vi "Simulation Kobuki Sensors.vi"(8 "error in":errorcluster, 9 "Feedback Input":T1, 10 "Robot":T2, 11 "simulator":T8={"configuration"={"maxTime"=5.0, "enableVisualization"=TRUE, "Environment Definition"=path "simulation configuration.ini", "Record Location"=path "Simulation Record.xml", "autograde?"=TRUE, "interactive?"=FALSE, "Feedback Mode"=enum."debug navigation", "Robot State Charts"=[path "C:/Users/blueuser/Desktop/Robo Sim Berkley/cpsgrader-release-0.4/Simulators/EECS149lab/src/LabVIEW/statechart/Simulation Statechart.vi"], "statechart"=path "iRobot Navigation State Machine.vi"}, "Statechart\ndisplay"=refnum, "first step?"=FALSE, "Robots Simulation Statecharts"=[], "Robots"=[]}) -> (0 "error out":errorcluster, 1 "Feedback Output":T1, 2 "sensors":T3 {"Kobuki Sensors"."Charger Source" items=["DISCHARGING"=0, "DOCKING_CHARGED"=2, "DOCKING_CHARGING"=6, "ADAPTER_CHARGED"=18, "ADAPTER_CHARGING"=22]; "accelerometer"."z axis (g)" format="%.3f"; "accelerometer"."y axis (g)" format="%.3f"; "accelerometer"."x axis (g)" format="%.3f"}, 3 "simulator":T8={"configuration"={"maxTime"=5.0, "enableVisualization"=TRUE, "Environment Definition"=path "simulation configuration.ini", "Record Location"=path "Simulation Record.xml", "autograde?"=TRUE, "interactive?"=FALSE, "Feedback Mode"=enum."debug navigation", "Robot State Charts"=[path "C:/Users/blueuser/Desktop/Robo Sim Berkley/cpsgrader-release-0.4/Simulators/EECS149lab/src/LabVIEW/statechart/Simulation Statechart.vi"], "statechart"=path "iRobot Navigation State Machine.vi"}, "Statechart\ndisplay"=refnum, "first step?"=FALSE, "Robots Simulation Statecharts"=[], "Robots"=[]})   [LabVIEW 2015]
doc: "Simulates iRobot sensors. Automatically accumulates distance and angle."
uses:
  Simulator.ctl
  <instrlib>/DC Motor Controller/HAIOL/DC Motor Controller.lvclass
  CyberSim interface/Simulation Configuration.ctl
  autograder/feedbackMode.ctl
  Multi Bot Code/RobotData.ctl
  shared/Sensors.ctl
  shared/Accelerometer.ctl
  Kobuki/KobukiSensors.ctl
  Kobuki/Kobuki Bumps and WheelDrops.ctl
  Kobuki/Kobuki Buttons.ctl
  Multi Bot Code/Sim Sensors Feedback.ctl
  <vilib>/Analysis/coordinate.llb/Angle Units.ctl
  <vilib>/Analysis/coordinate.llb/Wrap Angle (scalar).vi
  <vilib>/Analysis/BLAS.llb/dnrm2 - Vector 2-Norm (DBL).vi
  <resource>/objmgr/LVODE.rc
  <vilib>/Analysis/NI_AALBLAS.lvlib
  <vilib>/robotics/Kinematics/NI_Kinematics.lvlib
  <vilib>/Analysis/NI_AAL_Angle.lvlib
panel:
  out "size(s)":i32
  out "Roll":dbl
  out "pitch":dbl
  out "Yaw":dbl
  # "Electrical: charging, battery, OI mode"
  # "Sensors: bump, cliff, button, wheel drop"
  # "Motors:"
  # "Inertia"
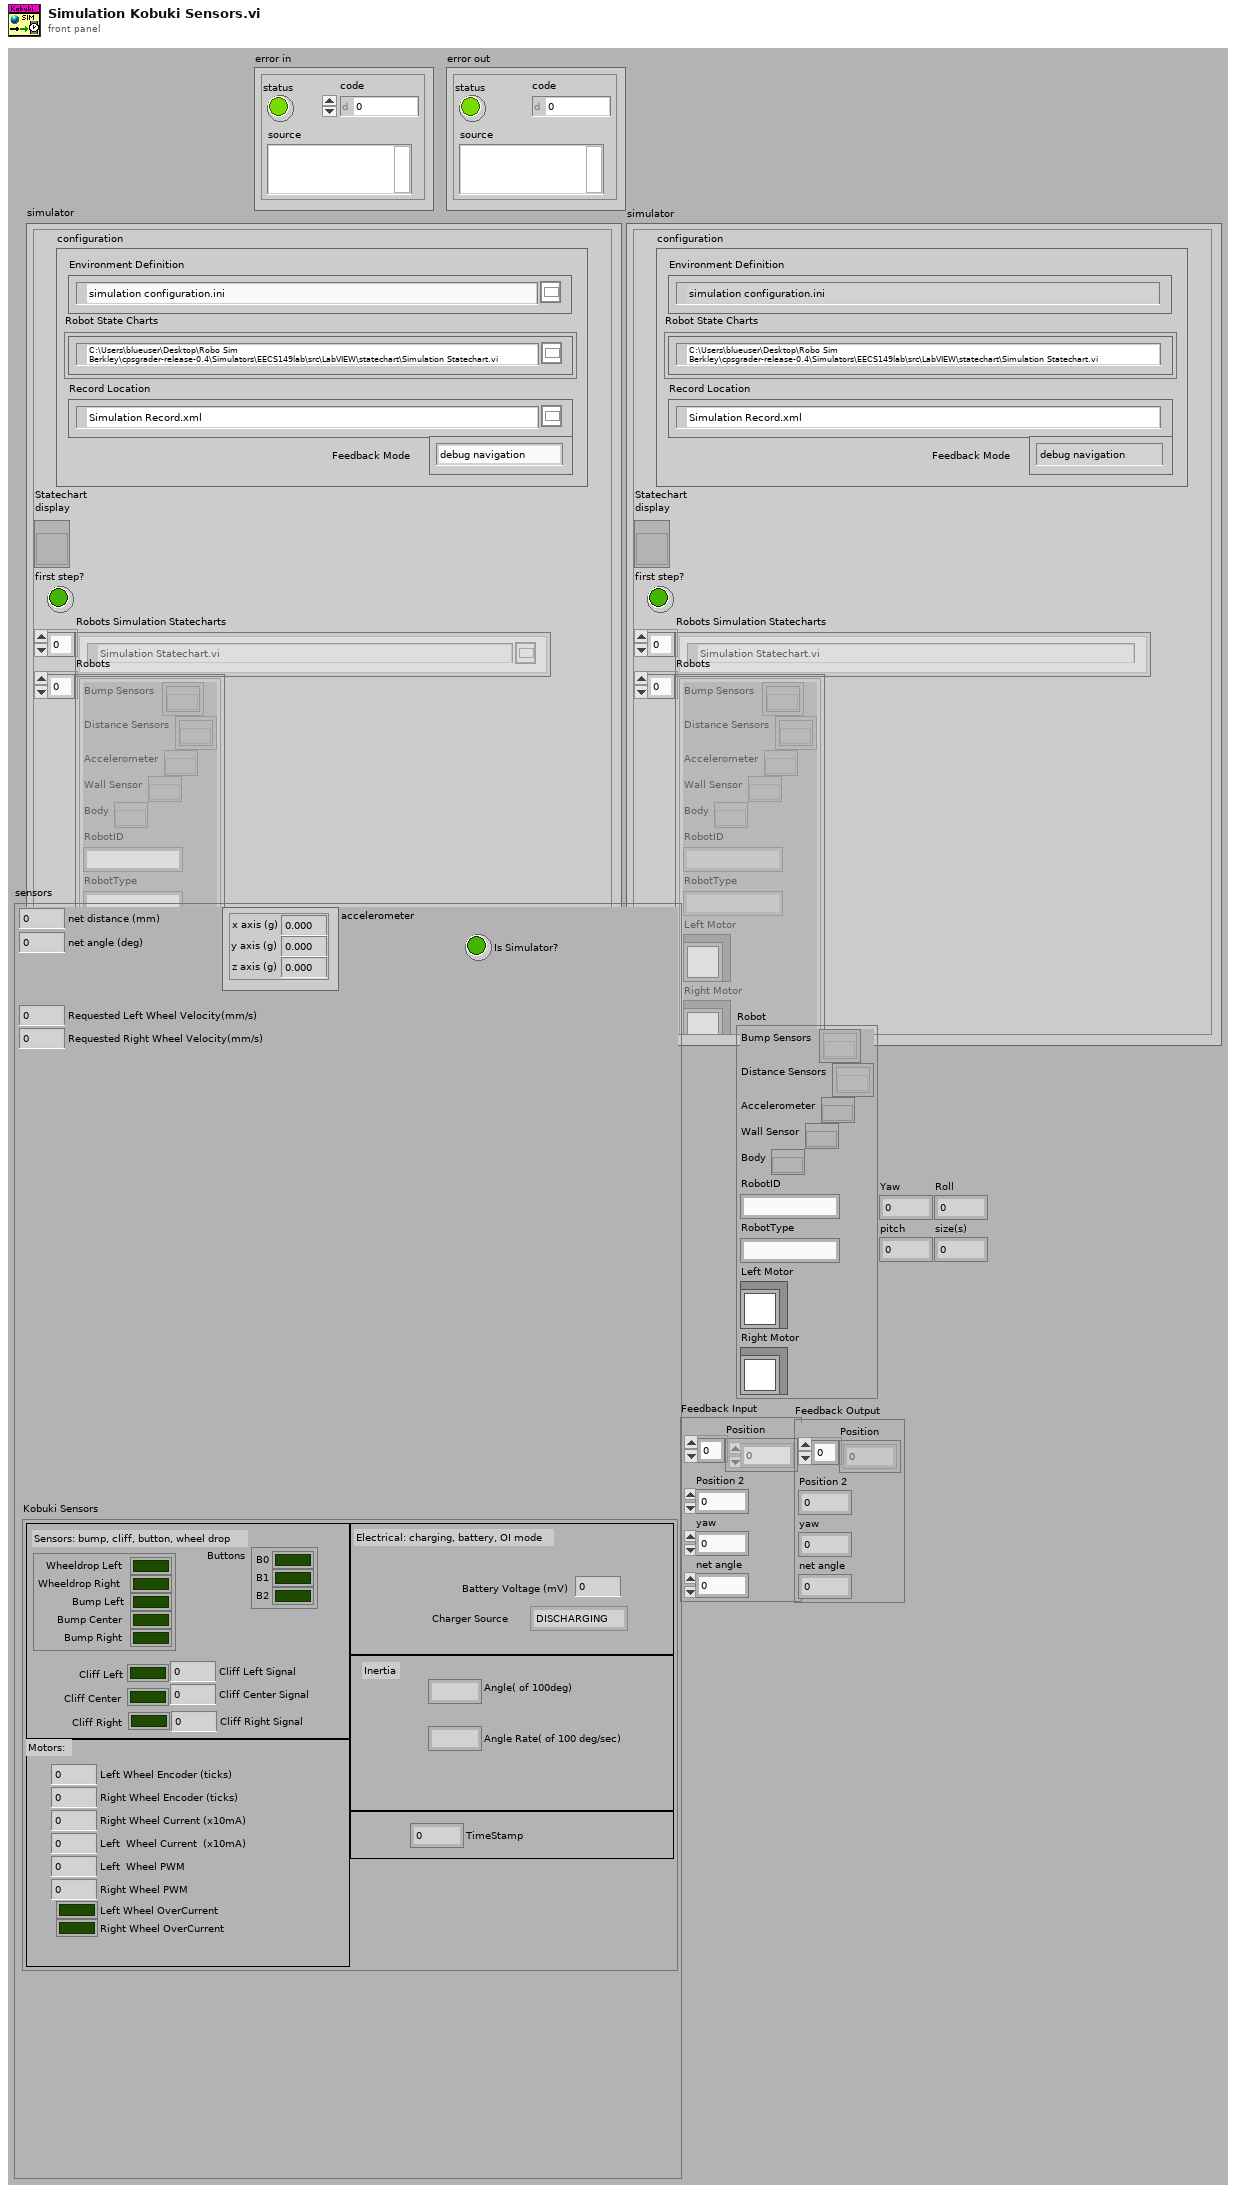
[diagram p1: front panel]
types:
  T1 = typedef "Sim Sensors Feedback.ctl" = cluster{"Position":sgl[], "Position 2":dbl, "yaw":dbl, "net angle":dbl}
  T2 = typedef "RobotData.ctl" = cluster{"Bump Sensors":refnum<k20>[], "Distance Sensors":refnum<k20>[], "Accelerometer":refnum<k20>, "Wall Sensor":refnum<k20>, "Body":refnum<k20>, "RobotID":string, "RobotType":string, "Left Motor":refnum<class "DC Motor Controller.lvclass">, "Right Motor":refnum<class "DC Motor Controller.lvclass">}
  T3 = typedef "Sensors.ctl" = cluster{"net distance (mm)":i32, "net angle (deg)":i32, "accelerometer":T4, "Is Simulator?":bool, "Kobuki Sensors":T5, "Requested Left Wheel Velocity(mm/s)":i32, "Requested Right Wheel Velocity(mm/s)":i32}
  T4 = typedef "Accelerometer.ctl" = cluster{"x axis (g)":dbl, "y axis (g)":dbl, "z axis (g)":dbl}
  T5 = typedef "KobukiSensors.ctl" = cluster{"Bumps + Wheel Drops":T6, "Cliff Left":bool, "Cliff Center":bool, "Cliff Right":bool, "Cliff Left Signal":u16, "Cliff Center Signal":u16, "Cliff Right Signal":u16, "Buttons":T7, "Left Wheel Encoder (ticks)":u16, "Right Wheel Encoder (ticks) ":u16, "Left  Wheel PWM":i8, "Right Wheel PWM":i8, "Left Wheel OverCurrent":bool, "Right Wheel OverCurrent ":bool, "Right Wheel Current (x10mA)":i16, "Left  Wheel Current  (x10mA)":i16, "TimeStamp":u16, "Battery Voltage (mV)":i16, "Angle( of 100deg)":i16, "Angle Rate( of 100 deg/sec)":i16, "Charger Source ":i8}
  T6 = typedef "Kobuki Bumps and WheelDrops.ctl" = cluster{"Wheeldrop Left":bool, "Wheeldrop Right":bool, "Bump Left":bool, "Bump Center":bool, "Bump Right":bool}
  T7 = typedef "Kobuki Buttons.ctl" = cluster{"B0":bool, "B1":bool, "B2":bool}
  T8 = typedef "Simulator.ctl" = cluster{"configuration":T9, "Statechart\ndisplay":refnum<vi>, "first step?":bool, "Robots Simulation Statecharts":path[], "Robots":T2[]}
  T9 = typedef "Simulation Configuration.ctl" = cluster{"maxTime":sgl, "enableVisualization":bool, "Environment Definition":path, "Record Location":path, "autograde?":bool, "interactive?":bool, "Feedback Mode":T10, "Robot State Charts":path[], "statechart":path}
  T10 = typedef "feedbackMode.ctl" = enum32{"debug navigation", "debug hill climb", "autograde navigation", "autograde hill climb"}
  T11 = typedef "NI_AAL_Angle.lvlib/Angle Units.ctl" = i32
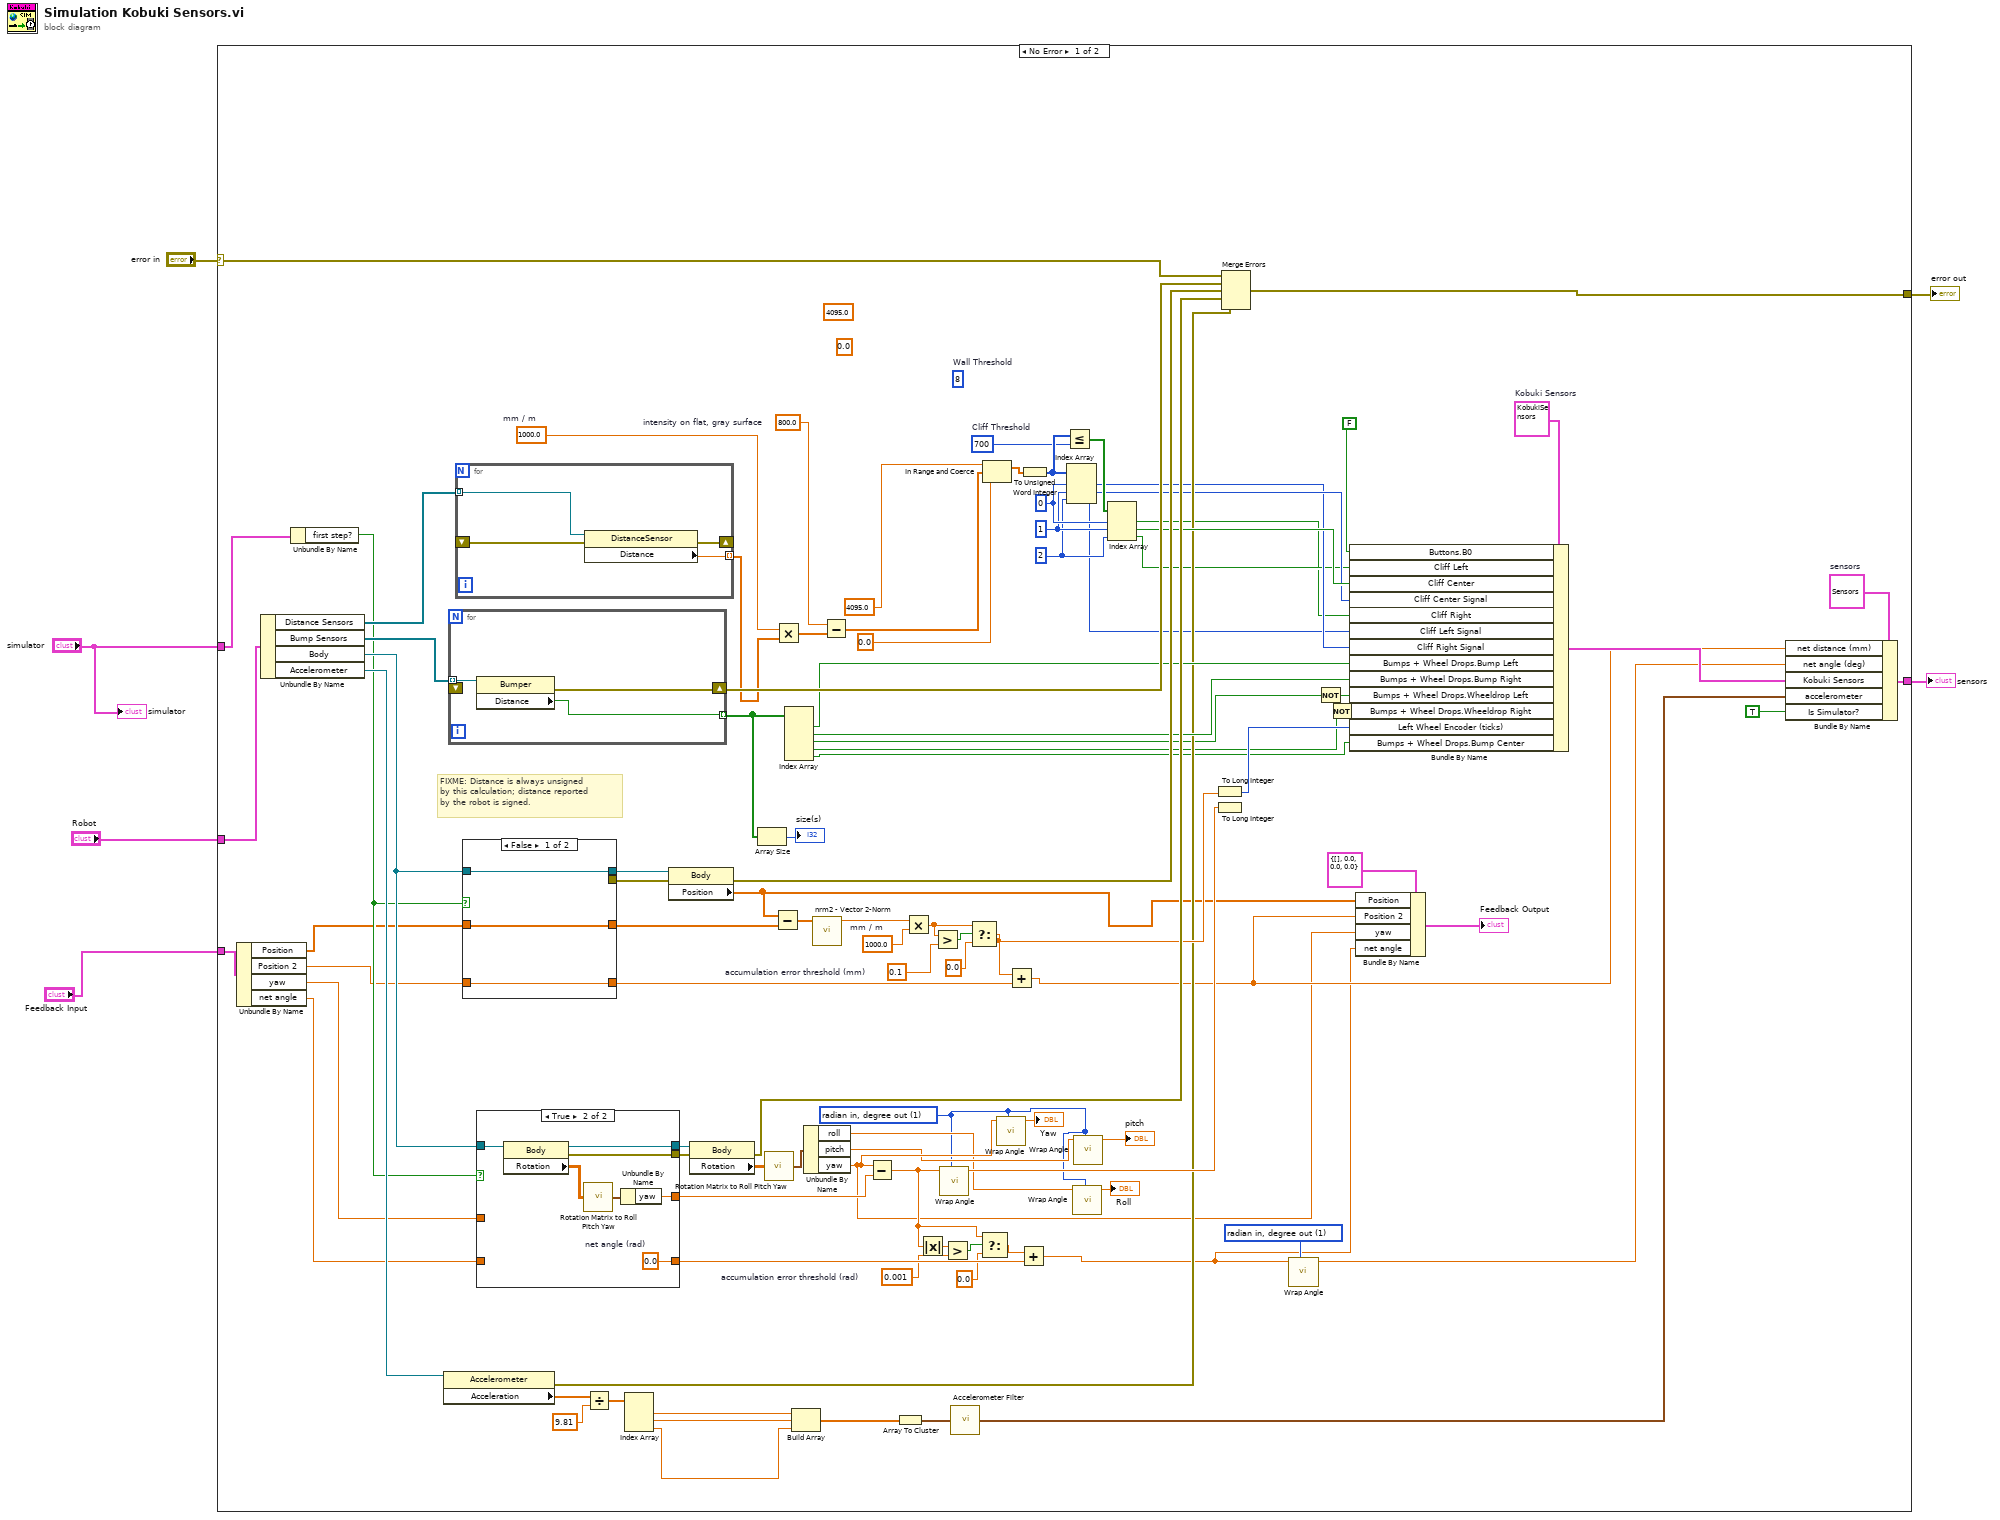
[diagram p0: block diagram]
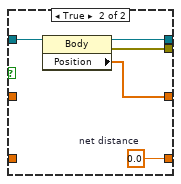
[diagram p3: hidden frame]
diagram:
  n1 = case shown="No Error" "error in" {
    selector: "error in" -> [w71 w134]
    tunnel: [w76 _] -> w6
    tunnel: "simulator" -> [w61 _]
    tunnel: [w72 w134] -> w4
    tunnel: "Robot" -> [w62 _]
    tunnel: "Feedback Input" -> [w59 _]
    frame No Error {
      w14 = T11 1 items=["radian in, radian out", "radian in, degree out", "degree in, degree out", "degree in, radian out"] ("angle units")
      w29 = 0.001  # accumulation error threshold (rad)
      w40 = 0.1  # accumulation error threshold (mm)
      w45 = 1000.0  # mm / m
      w24 = 2 ("index")
      w65 = 1 ("index")
      w66 = 0 ("index")
      w77 = T3 {"net distance (mm)"=0, "net angle (deg)"=0, "accelerometer"={"x axis (g)"=0.0, "y axis (g)"=0.0, "z axis (g)"=0.0}, "Is Simulator?"=FALSE, "Kobuki Sensors"={"Bumps + Wheel Drops"={"Wheeldrop Left"=FALSE, "Wheeldrop Right"=FALSE, "Bump Left"=FALSE, "Bump Center"=FALSE, "Bump Right"=FALSE}, "Cliff Left"=FALSE, "Cliff Center"=FALSE, "Cliff Right"=FALSE, "Cliff Left Signal"=0, "Cliff Center Signal"=0, "Cliff Right Signal"=0, "Buttons"={"B0"=FALSE, "B1"=FALSE, "B2"=FALSE}, "Left Wheel Encoder (ticks)"=0, "Right Wheel Encoder (ticks) "=0, "Left  Wheel PWM"=0, "Right Wheel PWM"=0, "Left Wheel OverCurrent"=FALSE, "Right Wheel OverCurrent "=FALSE, "Right Wheel Current (x10mA)"=0, "Left  Wheel Current  (x10mA)"=0, "TimeStamp"=0, "Battery Voltage (mV)"=0, "Angle( of 100deg)"=0, "Angle Rate( of 100 deg/sec)"=0, "Charger Source "=0}, "Requested Left Wheel Velocity(mm/s)"=0, "Requested Right Wheel Velocity(mm/s)"=0}  # sensors
      (unwired) 4095.0 ("upper limit")
      (unwired) 0.0 ("lower limit")
      (unwired) u16 8  # Wall Threshold
      w90 = 800.0  # intensity on flat, gray surface
      w93 = T11 1 items=["radian in, radian out", "radian in, degree out", "degree in, degree out", "degree in, radian out"] ("angle units")
      w94 = 700  # Cliff Threshold
      w103 = T5 {"Bumps + Wheel Drops"={"Wheeldrop Left"=FALSE, "Wheeldrop Right"=FALSE, "Bump Left"=FALSE, "Bump Center"=FALSE, "Bump Right"=FALSE}, "Cliff Left"=FALSE, "Cliff Center"=FALSE, "Cliff Right"=FALSE, "Cliff Left Signal"=0, "Cliff Center Signal"=0, "Cliff Right Signal"=0, "Buttons"={"B0"=FALSE, "B1"=FALSE, "B2"=FALSE}, "Left Wheel Encoder (ticks)"=0, "Right Wheel Encoder (ticks) "=0, "Left  Wheel PWM"=0, "Right Wheel PWM"=0, "Left Wheel OverCurrent"=FALSE, "Right Wheel OverCurrent "=FALSE, "Right Wheel Current (x10mA)"=0, "Left  Wheel Current  (x10mA)"=0, "TimeStamp"=0, "Battery Voltage (mV)"=0, "Angle( of 100deg)"=0, "Angle Rate( of 100 deg/sec)"=0, "Charger Source "=0}  # Kobuki Sensors
      w107 = 1000.0  # mm / m
      # "FIXME: Distance is always unsigned\nby this calculation; distance reported\nby the robot is signed."
      n2 = Unbundle By Name(w59) -> ("Position"=w58:sgl[], "Position 2"=w57:dbl, "yaw"=w56:dbl, "net angle"=w55:dbl)
      n3 = Unbundle By Name(w62) -> ("Distance Sensors"=w68:refnum<k20>[], "Bump Sensors"=w108:refnum<k20>[], "Body"=w92:refnum<k20>, "Accelerometer"=w85:refnum<k20>)
      n4 = Unbundle By Name(w61) -> ("first step?"=w60:bool)
      n5 = property class="Accelerometer"(reference=w85) -> (error out=w70:errorcluster, "Acceleration"=w84:sgl[])  [unwired: 1 in, 1 out]
      n6 = for {
        tunnel: w108 -> [w133] mode=indexing
        tunnel: [w132] -> w10 mode=indexing
        shift-right: [w131] -> w106
        shift-left: _ -> [_]
        n7 = property class="Bumper"(reference=w133) -> (error out=w131:errorcluster, "Distance"=w132:bool)  [unwired: 1 in, 1 out]
      }
      n8 = for {
        tunnel: [w130] -> w67 mode=indexing
        shift-right: [w129] -> _
        shift-left: _ -> [w127]
        tunnel: w68 -> [w128] mode=indexing
        n9 = property class="DistanceSensor"(reference=w128, error in=w127) -> (error out=w129:errorcluster, "Distance"=w130:sgl)  [unwired: 1 out]
      }
      n10 = case shown="False" w60 {
        tunnel: w92 -> [w120 w126]
        tunnel: [w121 w123] -> w47
        tunnel: w58 -> [w121 _]
        tunnel: [_ w125] -> w48
        tunnel: [w120 w124] -> w49
        tunnel: w57 -> [w119 _]
        tunnel: [w119 w122] -> w43
        frame False {
        }
        frame True {
          w122 = 0.0  # net distance
          n11 = property class="Body"(reference=w126) -> (reference out=w124:refnum<k20>, error out=w125:errorcluster, "Position"=w123:sgl[])  [unwired: 1 in]
        }
      }
      n12 = case shown="True" w60 {
        tunnel: w92 -> [w111 w118]
        tunnel: [w111 w117] -> w38
        tunnel: [_ w116] -> w37
        tunnel: [w110 w113] -> w34
        tunnel: w56 -> [w110 _]
        tunnel: [w109 w112] -> w31
        tunnel: w55 -> [w109 _]
        frame False {
        }
        frame True {
          w112 = 0.0  # net angle (rad)
          n13 = property class="Body"(reference=w118) -> (reference out=w117:refnum<k20>, error out=w116:errorcluster, "Rotation"=w115:sgl[][])  [unwired: 1 in]
          n14 = call <vilib>:"Rotation Matrix to Roll Pitch Yaw.vi"("rotation matrix"=w115) -> ("angles"=w114:cluster{"roll":dbl, "pitch":dbl, "yaw":dbl})
          n15 = Unbundle By Name(w114) -> ("yaw"=w113:dbl)
        }
      }
      n16 = Divide(x=w84, y=9.81) -> (x/y=w82:dbl[])
      n17 = Index Array(array=w82) -> (element #1=w12:dbl, element #2=w11:dbl, element #3=w81:dbl)  [unwired: 3 in]
      n18 = property class="Body"(reference=w49, error in=w48) -> (error out=w105:errorcluster, "Position"=w52:sgl[])  [unwired: 1 out]
      n19 = property class="Body"(reference=w38, error in=w37) -> (error out=w104:errorcluster, "Rotation"=w36:sgl[][])  [unwired: 1 out]
      n20 = Array Size(array=w10) -> (size(s)=→"size(s)":i32)
      n21 = call <vilib>:"Rotation Matrix to Roll Pitch Yaw.vi"("rotation matrix"=w36) -> ("angles"=w35:cluster{"roll":dbl, "pitch":dbl, "yaw":dbl})
      n22 = Subtract(x=w52, y=w47) -> (x-y=w44:sgl[])
      n23 = Multiply(x=w107, y=w67) -> (x*y=w91:dbl[])
      n24 = Index Array(array=w10) -> (element #1=w102:bool, element #2=w101:bool, element #3=w26:bool, element #4=w25:bool, element #5=w63:bool)  [unwired: 5 in]
      n25 = Build Array(w12, w11, w81) -> (w80:dbl[])
      n26 = Unbundle By Name(w35) -> ("roll"=w15:dbl, "pitch"=w17:dbl, "yaw"=w19:dbl)
      n27 = call-poly <vilib>:"nrm2 - Vector 2-Norm.vi"("x"=w44) -> ("dnrm2"=w46:dbl)  [unwired: 9 in, 1 out]
      n28 = Subtract(x=w90, y=w91) -> (x-y=w87:dbl[])
      n29 = Subtract(x=w19, y=w34) -> (x-y=w27:dbl)
      n30 = Array To Cluster(array=w80) -> (cluster=w74:cluster{"[0]":dbl, "[1]":dbl, "[2]":dbl})
      n31 = Multiply(x=w46, y=w45) -> (x*y=w42:dbl)
      n32 = Absolute Value(x=w27) -> (abs(x)=w28:dbl)
      n33 = Greater?(x=w42, y=w40) -> (0:w41:bool)
      n34 = call-poly <vilib>:"Wrap Angle.vi"("angle units"=w14, "angle in"=w27) -> ("angle out"=w98:dbl)  [unwired: 8 in, 1 out]
      n35 = Greater?(x=w28, y=w29) -> (0:w33:bool)
      n36 = call "Accelerometer Filter.vi"("accelerometer (g)"=w74) -> ("filtered accelerometer (g)"=w73:T4)  [unwired: 3 in]
      n37 = Select(t=w42, s=w41, f=0.0) -> (s? t:f=w99:dbl)
      n38 = Select(t=w27, s=w33, f=0.0) -> (s? t:f=w32:dbl)
      n39 = In Range and Coerce(upper limit=4095.0, x=w87, lower limit=0.0) -> (coerced(x)=w86:dbl[])  [unwired: 1 out]
      n40 = call-poly <vilib>:"Wrap Angle.vi"("angle units"=w14, "angle in"=w19) -> ("angle out"=→"Yaw":dbl)  [unwired: 8 in, 1 out]
      n41 = Add(x=w99, y=w43) -> (x+y=w51:dbl)
      n42 = Add(x=w32, y=w31) -> (x+y=w50:dbl)
      n43 = To Unsigned Word Integer(number=w86) -> (unsigned 16bit integer=w97:u16[])
      n44 = Less Or Equal?(x=w97, y=w94) -> (x <= y?=w96:bool[])
      n45 = Index Array(array=w97, index #1=w66, index #2=w65, index #3=w24) -> (element #1=w23:u16, element #2=w64:u16, element #3=w22:u16)
      n46 = call-poly <vilib>:"Wrap Angle.vi"("angle units"=w14, "angle in"=w15) -> ("angle out"=→"Roll":dbl)  [unwired: 8 in, 1 out]
      n47 = call-poly <vilib>:"Wrap Angle.vi"("angle units"=w14, "angle in"=w17) -> ("angle out"=→"pitch":dbl)  [unwired: 8 in, 1 out]
      n48 = Index Array(array=w96, index #1=w66, index #2=w65, index #3=w24) -> (element #1=w20:bool, element #2=w95:bool, element #3=w21:bool)
      n49 = To Long Integer(number=w99) -> (32bit integer=w100:i32)
      n50 = To Long Integer(number=w98) -> ()  [unwired: 1 out]
      n51 = Merge Errors(w71, w106, w105, w104, w70) -> (w72:errorcluster)
      n52 = call-poly <vilib>:"Wrap Angle.vi"("angle units"=w93, "angle in"=w50) -> ("angle out"=w78:dbl)  [unwired: 8 in, 1 out]
      n53 = Not(x=w26) -> (.not. x?=w8:bool)
      n54 = Not(x=w25) -> (.not. x?=w7:bool)
      n55 = Bundle By Name(cluster=w103, "Buttons.B0"=FALSE ("Buttons.Play"), "Cliff Left"=w21, "Cliff Center"=w95, "Cliff Center Signal"=w64, "Cliff Right"=w20, "Cliff Left Signal"=w22, "Cliff Right Signal"=w23, "Bumps + Wheel Drops.Bump Left"=w102, "Bumps + Wheel Drops.Bump Right"=w101, "Bumps + Wheel Drops.Wheeldrop Left"=w8, "Bumps + Wheel Drops.Wheeldrop Right"=w7, "Left Wheel Encoder (ticks)"=w100, "Bumps + Wheel Drops.Bump Center"=w63) -> (w79:T5)
      n56 = Bundle By Name(cluster=T1 {"Position"=[], "Position 2"=0.0, "yaw"=0.0, "net angle"=0.0} ("output cluster"), "Position"=w52, "Position 2"=w51, "yaw"=w19, "net angle"=w50) -> (→"Feedback Output":T1)
      n57 = Bundle By Name(cluster=w77, "net distance (mm)"=w51, "net angle (deg)"=w78, "Kobuki Sensors"=w79, "accelerometer"=w73, "Is Simulator?"=TRUE) -> (w76:T3)
    }
    frame Error {
    }
  }
  "error out" <- w4
  "sensors" <- w6
  "simulator" <- "simulator"
